vi "Get Experiment.vi"(8 "error in (no error)":errorcluster, 10 "id":u32, 11 "eLab in":refnum<class "PL eLabFTW Client.lvclass">) -> (0 "error out":errorcluster, 2 "experiment":T1 {"steps"."finish datetime" format="%<%X\n%x>T"; "steps"."deadline datetime" format="%<%X\n%x>T"; "files"."creation datetime" format="%<%X\n%x>T"; "last change"."datetime" format="%<%X\n%x>T"; "start datetime" format="%<%X\n%x>T"; "creation datetime" format="%<%X\n%x>T"; "last comment"."datetime" format="%<%X\n%x>T"; "timestamp"."datetime" format="%<%X\n%x>T"; "lock"."datetime" format="%<%X\n%x>T"}, 3 "eLab out":refnum<class "PL eLabFTW Client.lvclass">)   [LabVIEW 2015, in "PL eLabFTW Client.lvclass"]
doc: "Gets experiment with the specified id."
uses:
  PL eLabFTW Client.lvclass
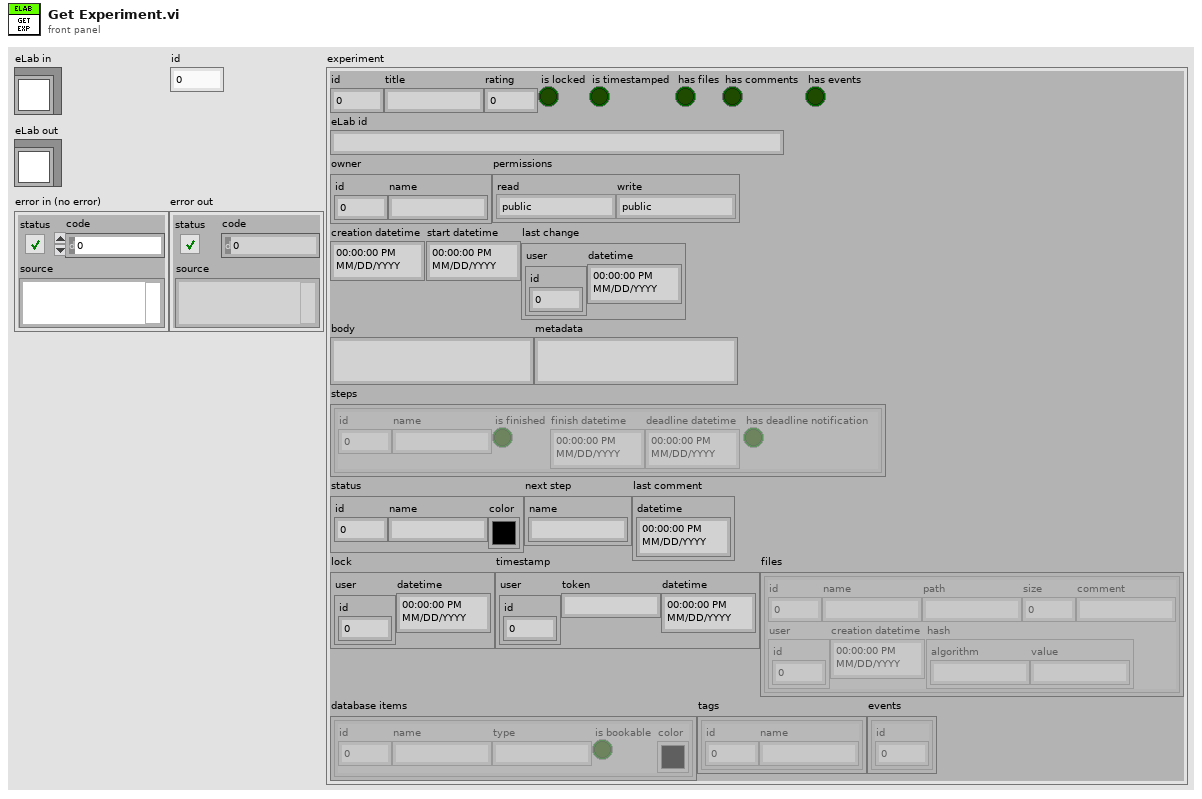
[diagram p1: front panel]
types:
  T1 = cluster{"id":u32, "title":string, "rating":u32, "is locked":bool, "is timestamped":bool, "has files":bool, "has comments":bool, "has events":bool, "eLab id":string, "owner":cluster{"id":u32, "name":string}, "permissions":cluster{"read":enum16{"public", "organization", "team", "owner and admins", "owner"}, "write":enum16{"public", "organization", "team", "owner and admins", "owner"}}, "creation datetime":timestamp, "start datetime":timestamp, "last change":cluster{"user":cluster{"id":u32}, "datetime":timestamp}, "body":string, "metadata":string, "steps":cluster{"id":u32, "name":string, "is finished":bool, "finish datetime":timestamp, "deadline datetime":timestamp, "has deadline notification":bool}[], "status":cluster{"id":u32, "name":string, "color":u32}, "next step":cluster{"name":string}, "last comment":cluster{"datetime":timestamp}, "lock":cluster{"user":cluster{"id":u32}, "datetime":timestamp}, "timestamp":cluster{"user":cluster{"id":u32}, "token":string, "datetime":timestamp}, "files":cluster{"id":u32, "name":string, "path":string, "size":u32, "comment":string, "user":cluster{"id":u32}, "creation datetime":timestamp, "hash":cluster{"algorithm":string, "value":string}}[], "database items":cluster{"id":u32, "name":string, "type":string, "is bookable":bool, "color":u32}[], "tags":cluster{"id":u32, "name":string}[], "events":cluster{"id":u32}[]}
  T2 = cluster{"id":string, "title":string, "date":string, "body":string, "category":string, "userid":string, "elabid":string, "locked":string, "lockedby":string, "lockedwhen":string, "timestamped":string, "timestampedby":string, "timestamptoken":string, "timestampedwhen":string, "canread":string, "canwrite":string, "datetime":string, "lastchange":string, "metadata":string, "rating":string, "lastchangeby":string, "state":string, "is_bound":string, "events_item_id":string, "events_id":string, "up_item_id":string, "has_attachment":string, "next_step":string, "category_id":string, "color":string, "fullname":string, "recent_comment":string, "has_comment":string, "tags":string, "tags_id":string, "uploads":cluster{"id":string, "real_name":string, "long_name":string, "comment":string, "item_id":string, "userid":string, "type":string, "created_at":string, "hash":string, "hash_algorithm":string, "storage":string, "filesize":string, "state":string}[], "links":cluster{"itemid":string, "title":string, "name":string, "bookable":string, "color":string}[], "steps":cluster{"id":string, "item_id":string, "body":string, "ordering":string, "finished":string, "finished_time":string, "deadline":string, "deadline_notif":string}[]}
  T3 = cluster{"id":i32, "title":i32, "date":i32, "body":i32, "category":i32, "userid":i32, "elabid":i32, "locked":i32, "lockedby":i32, "lockedwhen":i32, "timestamped":i32, "timestampedby":i32, "timestamptoken":i32, "timestampedwhen":i32, "canread":i32, "canwrite":i32, "datetime":i32, "lastchange":i32, "metadata":i32, "rating":i32, "lastchangeby":i32, "state":i32, "is_bound":i32, "events_item_id":i32, "events_id":i32, "up_item_id":i32, "has_attachment":i32, "next_step":i32, "category_id":i32, "color":i32, "fullname":i32, "recent_comment":i32, "has_comment":i32, "tags":i32, "tags_id":i32, "uploads":cluster{"id":i32, "real_name":i32, "long_name":i32, "comment":i32, "item_id":i32, "userid":i32, "type":i32, "created_at":i32, "hash":i32, "hash_algorithm":i32, "storage":i32, "filesize":i32, "state":i32}[], "links":cluster{"itemid":i32, "title":i32, "name":i32, "bookable":i32, "color":i32}[], "steps":cluster{"id":i32, "item_id":i32, "body":i32, "ordering":i32, "finished":i32, "finished_time":i32, "deadline":i32, "deadline_notif":i32}[]}
  T4 = cluster{"id":string, "item_id":string, "body":string, "ordering":string, "finished":string, "finished_time":string, "deadline":string, "deadline_notif":string}[]
  T5 = cluster{"id":string, "real_name":string, "long_name":string, "comment":string, "item_id":string, "userid":string, "type":string, "created_at":string, "hash":string, "hash_algorithm":string, "storage":string, "filesize":string, "state":string}[]
  T6 = cluster{"itemid":string, "title":string, "name":string, "bookable":string, "color":string}[]
  T7 = cluster{"id":bool, "title":bool, "date":bool, "body":bool, "category":bool, "userid":bool, "elabid":bool, "locked":bool, "lockedby":bool, "lockedwhen":bool, "timestamped":bool, "timestampedby":bool, "timestamptoken":bool, "timestampedwhen":bool, "canread":bool, "canwrite":bool, "datetime":bool, "lastchange":bool, "metadata":bool, "rating":bool, "lastchangeby":bool, "state":bool, "is_bound":bool, "events_item_id":bool, "events_id":bool, "up_item_id":bool, "has_attachment":bool, "next_step":bool, "category_id":bool, "color":bool, "fullname":bool, "recent_comment":bool, "has_comment":bool, "tags":bool, "tags_id":bool, "uploads":cluster{"id":bool, "real_name":bool, "long_name":bool, "comment":bool, "item_id":bool, "userid":bool, "type":bool, "created_at":bool, "hash":bool, "hash_algorithm":bool, "storage":bool, "filesize":bool, "state":bool}[], "links":cluster{"itemid":bool, "title":bool, "name":bool, "bookable":bool, "color":bool}[], "steps":cluster{"id":bool, "item_id":bool, "body":bool, "ordering":bool, "finished":bool, "finished_time":bool, "deadline":bool, "deadline_notif":bool}[]}
  T8 = cluster{"id":i32, "item_id":i32, "body":i32, "ordering":i32, "finished":i32, "finished_time":i32, "deadline":i32, "deadline_notif":i32}
  T9 = cluster{"id":bool, "item_id":bool, "body":bool, "ordering":bool, "finished":bool, "finished_time":bool, "deadline":bool, "deadline_notif":bool}
  T10 = cluster{"id":u32, "name":string, "is finished":bool, "finish datetime":timestamp, "deadline datetime":timestamp, "has deadline notification":bool}
  T11 = cluster{"id":i32, "real_name":i32, "long_name":i32, "comment":i32, "item_id":i32, "userid":i32, "type":i32, "created_at":i32, "hash":i32, "hash_algorithm":i32, "storage":i32, "filesize":i32, "state":i32}
  T12 = cluster{"id":u32, "name":string, "path":string, "size":u32, "comment":string, "user":cluster{"id":u32}, "creation datetime":timestamp, "hash":cluster{"algorithm":string, "value":string}}
  T13 = cluster{"itemid":i32, "title":i32, "name":i32, "bookable":i32, "color":i32}
  T14 = cluster{"itemid":bool, "title":bool, "name":bool, "bookable":bool, "color":bool}
  T15 = cluster{"id":u32, "name":string, "type":string, "is bookable":bool, "color":u32}
  T16 = enum16{"public", "organization", "team", "owner and admins", "owner"}
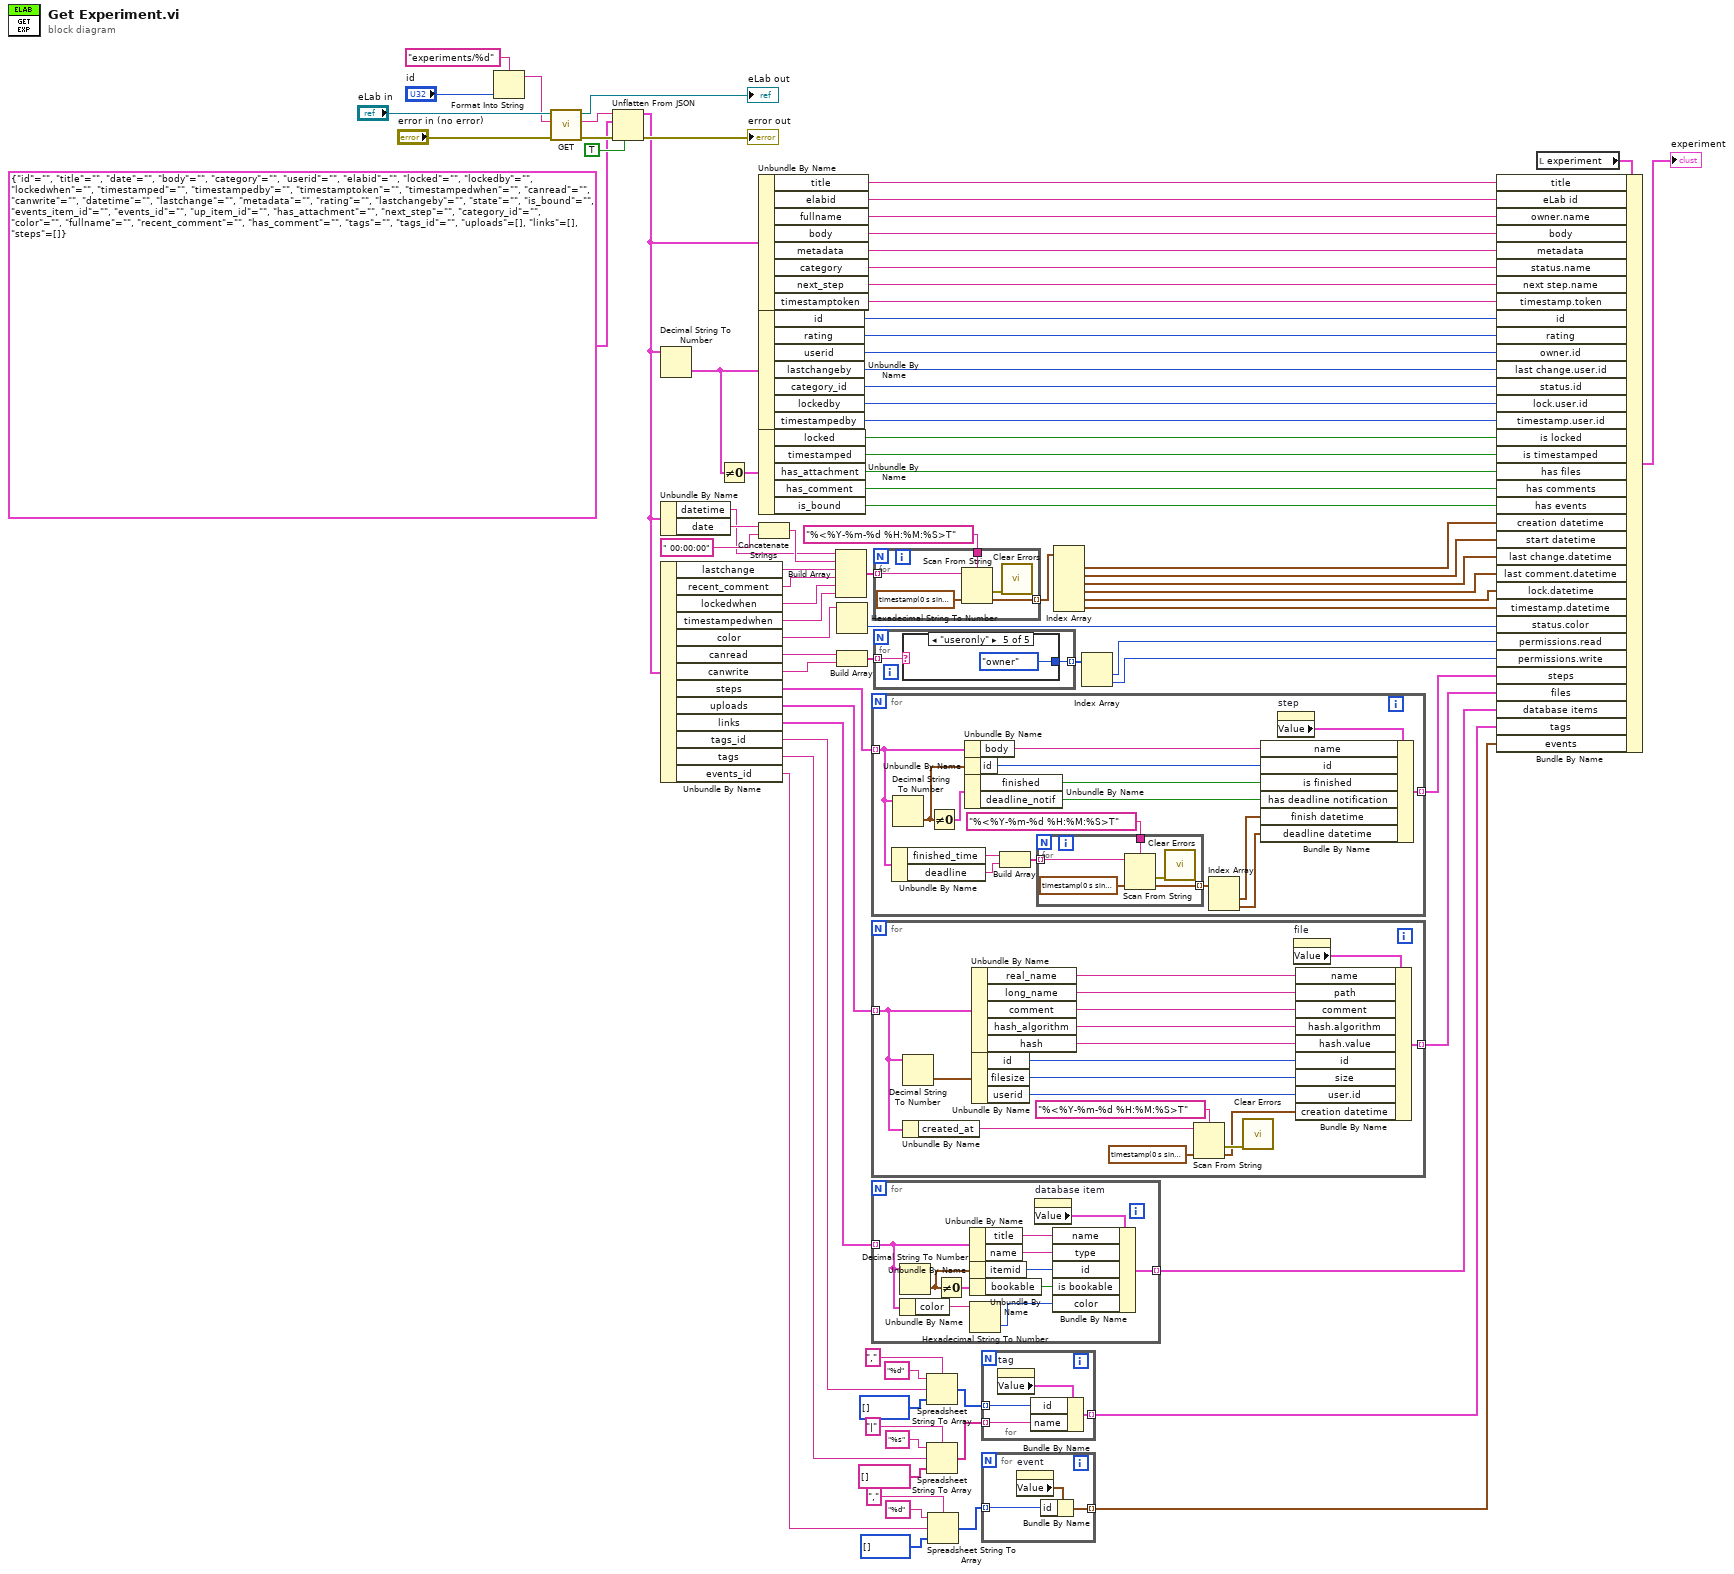
[diagram p0: block diagram]
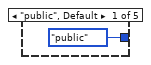
[diagram p2: hidden frame]
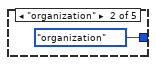
[diagram p3: hidden frame]
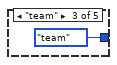
[diagram p4: hidden frame]
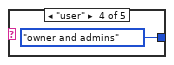
[diagram p5: hidden frame]
diagram:
  n1 = Format Into String(format string="experiments/%d", "id") -> (resulting string=w76:string)  [unwired: 2 in, 1 out]
  n2 = call "GET.vi"("error in (no error)"="error in (no error)", "relative URL"=w76, "eLab in"="eLab in") -> ("error out"=w81:errorcluster, "response body"=w79:string, "eLab out"=→"eLab out":refnum<class "PL eLabFTW Client.lvclass">)  [unwired: 6 in]
  n3 = Unflatten From JSON(JSON string=w79, type and defaults=T2 {"id"="", "title"="", "date"="", "body"="", "category"="", "userid"="", "elabid"="", "locked"="", "lockedby"="", "lockedwhen"="", "timestamped"="", "timestampedby"="", "timestamptoken"="", "timestampedwhen"="", "canread"="", "canwrite"="", "datetime"="", "lastchange"="", "metadata"="", "rating"="", "lastchangeby"="", "state"="", "is_bound"="", "events_item_id"="", "events_id"="", "up_item_id"="", "has_attachment"="", "next_step"="", "category_id"="", "color"="", "fullname"="", "recent_comment"="", "has_comment"="", "tags"="", "tags_id"="", "uploads"=[], "links"=[], "steps"=[]}, default null elements? (F)=TRUE, error in (no error)=w81) -> (value=w25:T2, error out=→"error out":errorcluster)  [unwired: 3 in]
  n4 = Decimal String To Number(string=w25) -> (number=w65:T3)  [unwired: 2 in, 1 out]
  n5 = Unbundle By Name(w25) -> ("datetime"=w40:string, "date"=w43:string)
  n6 = Unbundle By Name(w25) -> ("lastchange"=w58:string, "recent_comment"=w59:string, "lockedwhen"=w35:string, "timestampedwhen"=w36:string, "color"=w53:string, "canread"=w51:string, "canwrite"=w50:string, "steps"=w23:T4, "uploads"=w21:T5, "links"=w19:T6, "tags_id"=w10:string, "tags"=w9:string, "events_id"=w7:string)
  n7 = Not Equal To 0?(x=w65) -> (x != 0?=w64:T7)
  n8 = Unbundle By Name(w25) -> ("title"=w73:string, "elabid"=w37:string, "fullname"=w72:string, "body"=w38:string, "metadata"=w32:string, "category"=w71:string, "next_step"=w70:string, "timestamptoken"=w31:string)
  n9 = Unbundle By Name(w65) -> ("id"=w69:i32, "rating"=w68:i32, "userid"=w67:i32, "lastchangeby"=w26:i32, "category_id"=w66:i32, "lockedby"=w30:i32, "timestampedby"=w29:i32)
  n10 = Unbundle By Name(w64) -> ("locked"=w63:bool, "timestamped"=w62:bool, "has_attachment"=w61:bool, "has_comment"=w60:bool, "is_bound"=w1:bool)
  n11 = Concatenate Strings(w43, " 00:00:00" ("string")) -> (w42:string)
  n12 = Build Array(w40, w42, w58, w59, w35, w36) -> (w57:string[])
  n13 = Hexadecimal String To Number(string=w53) -> (number=w52:u32)  [unwired: 2 in, 1 out]
  n14 = Build Array(w51, w50) -> (w49:string[])
  n15 = for {
    tunnel: [w99] -> w24 mode=indexing
    tunnel: w23 -> [w92] mode=indexing
    n16 = Unbundle By Name(w92) -> ("finished_time"=w90:string, "deadline"=w89:string)
    n17 = Decimal String To Number(string=w92) -> (number=w96:T8)  [unwired: 2 in, 1 out]
    n18 = Not Equal To 0?(x=w96) -> (x != 0?=w95:T9)
    n19 = Unbundle By Name(w92) -> ("body"=w98:string)
    n20 = Unbundle By Name(w96) -> ("id"=w97:i32)
    n21 = Unbundle By Name(w95) -> ("finished"=w94:bool, "deadline_notif"=w93:bool)
    n22 = Build Array(w90, w89) -> (w88:string[])
    n23 = for {
      tunnel: w88 -> [w103] mode=indexing
      tunnel: [w102] -> w87 mode=indexing
      tunnel: "%<%Y-%m-%d %H:%M:%S>T" ("format string") -> [w101]
      n24 = Scan From String(format string=w101, input string=w103, default 1=timestamp(0 s since 1904-01-01) ("from")) -> (error out=w105:errorcluster, output 1=w102:timestamp)  [unwired: 2 in, 2 out]
      n25 = call <vilib>:"Clear Errors.vi"("error in (no error)"=w105) -> ()  [unwired: 5 in, 2 out]
    }
    n26 = Index Array(array=w87) -> (element #1=w86:timestamp, element #2=w85:timestamp)  [unwired: 2 in]
    n27 = property on="step" class="Clust (strict)"() -> ("Value"=w100:T10)  [unwired: 2 in, 2 out]
    n28 = Bundle By Name(cluster=w100, "name"=w98, "id"=w97, "is finished"=w94, "has deadline notification"=w93, "finish datetime"=w86, "deadline datetime"=w85) -> (w99:T10)
  }
  n29 = for {
    tunnel: [w121] -> w22 mode=indexing
    tunnel: w21 -> [w107] mode=indexing
    n30 = Decimal String To Number(string=w107) -> (number=w115:T11)  [unwired: 2 in, 1 out]
    n31 = Unbundle By Name(w107) -> ("created_at"=w108:string)
    n32 = Unbundle By Name(w107) -> ("real_name"=w120:string, "long_name"=w119:string, "comment"=w118:string, "hash_algorithm"=w117:string, "hash"=w116:string)
    n33 = Unbundle By Name(w115) -> ("id"=w112:i32, "filesize"=w113:i32, "userid"=w114:i32)
    n34 = Scan From String(format string="%<%Y-%m-%d %H:%M:%S>T", input string=w108, default 1=timestamp(0 s since 1904-01-01) ("from")) -> (error out=w110:errorcluster, output 1=w106:timestamp)  [unwired: 2 in, 2 out]
    n35 = call <vilib>:"Clear Errors.vi"("error in (no error)"=w110) -> ()  [unwired: 5 in, 2 out]
    n36 = property on="file" class="Clust (strict)"() -> ("Value"=w122:T12)  [unwired: 2 in, 2 out]
    n37 = Bundle By Name(cluster=w122, "name"=w120, "path"=w119, "comment"=w118, "hash.algorithm"=w117, "hash.value"=w116, "id"=w112, "size"=w113, "user.id"=w114, "creation datetime"=w106) -> (w121:T12)
  }
  n38 = for {
    tunnel: [w132] -> w20 mode=indexing
    tunnel: w19 -> [w127] mode=indexing
    n39 = Decimal String To Number(string=w127) -> (number=w130:T13)  [unwired: 2 in, 1 out]
    n40 = Unbundle By Name(w127) -> ("color"=w124:string)
    n41 = Not Equal To 0?(x=w130) -> (x != 0?=w131:T14)
    n42 = Unbundle By Name(w127) -> ("title"=w129:string, "name"=w128:string)
    n43 = Unbundle By Name(w130) -> ("itemid"=w126:i32)
    n44 = Unbundle By Name(w131) -> ("bookable"=w125:bool)
    n45 = Hexadecimal String To Number(string=w124) -> (number=w123:u32)  [unwired: 2 in, 1 out]
    n46 = property on="database item" class="Clust (strict)"() -> ("Value"=w133:T15)  [unwired: 2 in, 2 out]
    n47 = Bundle By Name(cluster=w133, "name"=w129, "type"=w128, "id"=w126, "is bookable"=w125, "color"=w123) -> (w132:T15)
  }
  n48 = for {
    tunnel: w57 -> [w136] mode=indexing
    tunnel: [w135] -> w56 mode=indexing
    tunnel: "%<%Y-%m-%d %H:%M:%S>T" ("format string") -> [w134]
    n49 = Scan From String(format string=w134, input string=w136, default 1=timestamp(0 s since 1904-01-01) ("from")) -> (error out=w138:errorcluster, output 1=w135:timestamp)  [unwired: 2 in, 2 out]
    n50 = call <vilib>:"Clear Errors.vi"("error in (no error)"=w138) -> ()  [unwired: 5 in, 2 out]
  }
  n51 = for {
    tunnel: w49 -> [w140] mode=indexing
    tunnel: [w139] -> w48 mode=indexing
    n52 = case shown="\"useronly\"" w140 {
      tunnel: [T16."public" ("permissions.read") T16."organization" ("permissions.read") T16."team" ("permissions.read") T16."owner and admins" ("permissions.read") T16."owner" ("permissions.read")] -> w139
      frame "public", Default {
      }
      frame "organization" {
      }
      frame "team" {
      }
      frame "user" {
      }
      frame "useronly" {
      }
    }
  }
  n53 = Spreadsheet String To Array(delimiter (Tab)=",", format string="%d", spreadsheet string=w10, array type (2D Dbl)=u32[] []) -> (array=w6:u32[])
  n54 = Spreadsheet String To Array(delimiter (Tab)="|", format string="%s", spreadsheet string=w9, array type (2D Dbl)=string[] []) -> (array=w5:string[])
  n55 = Spreadsheet String To Array(delimiter (Tab)=",", format string="%d", spreadsheet string=w7, array type (2D Dbl)=u32[] []) -> (array=w3:u32[])
  n56 = for {
    tunnel: [w148] -> w4 mode=indexing
    tunnel: w6 -> [w147] mode=indexing
    tunnel: w5 -> [w146] mode=indexing
    n57 = property on="tag" class="Clust (strict)"() -> ("Value"=w149:cluster{"id":u32, "name":string})  [unwired: 2 in, 2 out]
    n58 = Bundle By Name(cluster=w149, "id"=w147, "name"=w146) -> (w148:cluster{"id":u32, "name":string})
  }
  n59 = for {
    tunnel: [w151] -> w2 mode=indexing
    tunnel: w3 -> [w150] mode=indexing
    n60 = property on="event" class="Clust (strict)"() -> ("Value"=w152:cluster{"id":u32})  [unwired: 2 in, 2 out]
    n61 = Bundle By Name(cluster=w152, "id"=w150) -> (w151:cluster{"id":u32})
  }
  n62 = Index Array(array=w56) -> (element #1=w39:timestamp, element #2=w44:timestamp, element #3=w55:timestamp, element #4=w54:timestamp, element #5=w33:timestamp, element #6=w34:timestamp)  [unwired: 6 in]
  n63 = Index Array(array=w48) -> (element #1=w47:T16, element #2=w46:T16)  [unwired: 2 in]
  n64 = local read "experiment"() -> (w28:T1)
  n65 = Bundle By Name(cluster=w28, "title"=w73, "eLab id"=w37, "owner.name"=w72, "body"=w38, "metadata"=w32, "status.name"=w71, "next step.name"=w70, "timestamp.token"=w31, "id"=w69, "rating"=w68, "owner.id"=w67, "last change.user.id"=w26, "status.id"=w66, "lock.user.id"=w30, "timestamp.user.id"=w29, "is locked"=w63, "is timestamped"=w62, "has files"=w61, "has comments"=w60, "has events"=w1, "creation datetime"=w39, "start datetime"=w44, "last change.datetime"=w55, "last comment.datetime"=w54, "lock.datetime"=w33, "timestamp.datetime"=w34, "status.color"=w52, "permissions.read"=w47, "permissions.write"=w46, "steps"=w24, "files"=w22, "database items"=w20, "tags"=w4, "events"=w2) -> (→"experiment":T1)
